vi "UnitTest-LogicFindingSizeMultiples.vi"(8 "error in (no error)":errorcluster, 10 "File Size":i32, 11 "DB Multiples Size":i32) -> (0 "error out":errorcluster, 3 "Limits":i32[](array[numeric]))   [LabVIEW 2014]
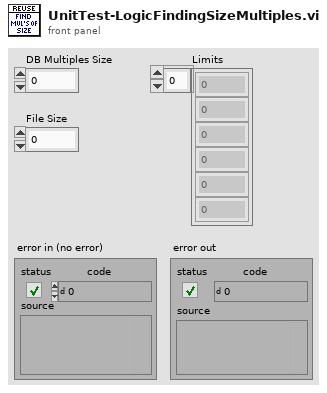
[diagram p1: front panel]
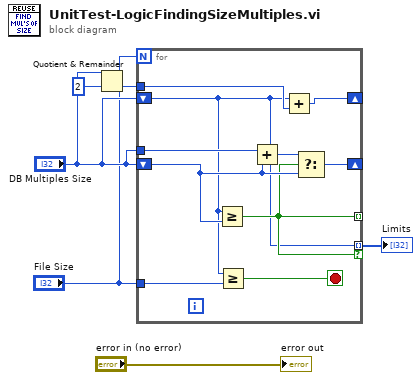
[diagram p0: block diagram]
diagram:
  n1 = Quotient & Remainder(x="DB Multiples Size", y=2) -> (floor(x/y)=w2:i32)  [unwired: 1 out]
  n2 = for {
    N: "File Size" -> [_]
    shift-right: [w13] -> _
    shift-left: "DB Multiples Size" -> [w9]
    shift-right: [w11] -> _
    shift-left: "DB Multiples Size" -> [w14]
    tunnel: "DB Multiples Size" -> [w15]
    tunnel: [w12] -> _ mode=indexing
    tunnel: [w9] -> w6 mode=indexing if=w12
    tunnel: w2 -> [w10]
    tunnel: "File Size" -> [w8]
    stop <- w7 stop-if-true
    n3 = Greater Or Equal?(x=w9, y=w14) -> (x >= y?=w12:bool)
    n4 = Greater Or Equal?(x=w9, y=w8) -> (x >= y?=w7:bool)
    n5 = Add(x=w15, y=w14) -> (x+y=w16:i32)
    n6 = Add(x=w9, y=w10) -> (x+y=w13:i32)
    n7 = Select(t=w16, s=w12, f=w14) -> (s? t:f=w11:i32)
  }
  "Limits" <- w6
  "error out" <- "error in (no error)"
